vi "Report Loop.vi"(8 "error in (no error)":errorcluster) -> (0 "error out":errorcluster)   [LabVIEW 2020, in "Report.lvlib"]
doc: "Message loop for handling messages pertaining to the acquisition of data from the hardware."
uses:
  Report.lvlib
  support/PCT FGV CMD.ctl
  REP Configuration.ctl
  Test Setting.ctl
  Acquisition State.ctl
  support/Message Queue/Enqueue Message (Single).vi
  <vilib>/Utility/error.llb/Error Cluster From Error Code.vi
  <vilib>/ErrorRing/Error Ring.xnode
  support/Message Queue/Message Queue.lvlib
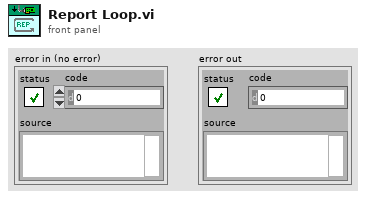
[diagram p1: front panel]
types:
  T1 = typedef "PCT FGV CMD.ctl" = enum16{"INIT", "GET", "SET"}
  T2 = typedef "Message Queue.lvlib/All Message Queues.ctl" = cluster{"UI":refnum<queue>, "Logging":refnum<queue>, "LOG":refnum<queue>, "ALARM":refnum<queue>, "Test":refnum<queue>, "Answer":refnum<queue>, "PLC":refnum<queue>, "DB":refnum<queue>, "Report":refnum<queue>, "OPC":refnum<queue>, "Procedure":refnum<queue>, "PalmSens":refnum<queue>, "SYS 7000 Reader":refnum<queue>, "SWITCH":refnum<queue>, "MOTOR":refnum<queue>, "MOTION":refnum<queue>, "HIDEN":refnum<queue>, "VALVE":refnum<queue>, "MFC":refnum<queue>, "PUMP IN":refnum<queue>, "PUMP OUT":refnum<queue>}
  T3 = typedef "Report.lvlib/REP Configuration.ctl" = cluster{"Test Setting":T4, "Measurements":string[][], "LOG REF":refnum<vi>, "Report Template":path, "Save Report path":path, "Data File Path":path, "Popup Dialog":bool}
  T4 = typedef "Report.lvlib/Test Setting.ctl" = cluster{"Test_Num":i32, "Test_ID":i32, "Proc_ID":i32, "Max Force":dbl, "User":string, "SN":string, "Date":string}
  T5 = typedef "Report.lvlib/Acquisition State.ctl" = enum16{"Idle", "Acquiring"}
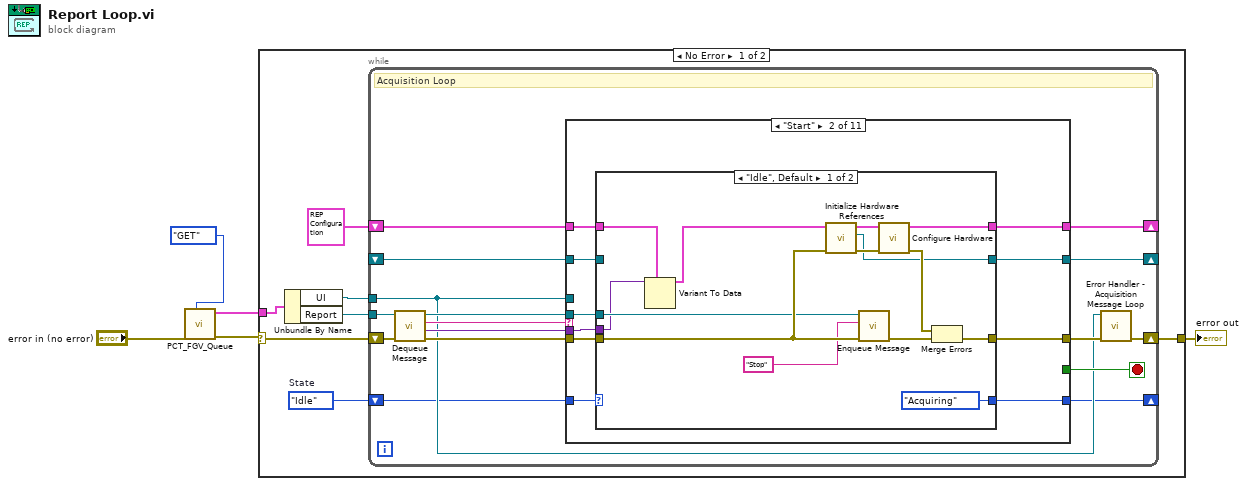
[diagram p0: block diagram]
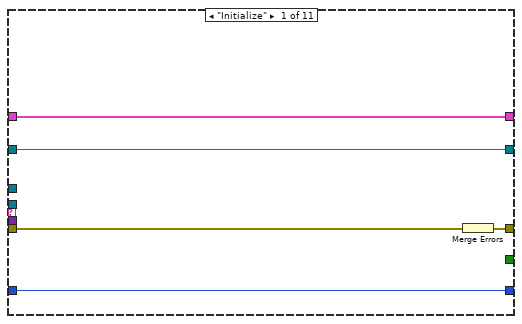
[diagram p2: hidden frame]
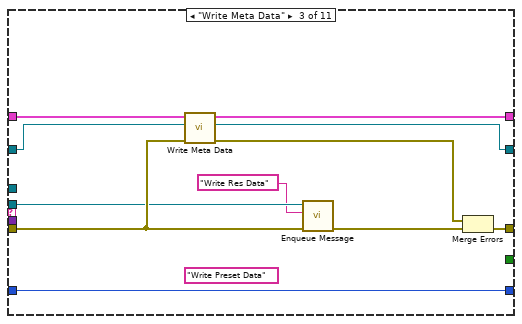
[diagram p4: hidden frame]
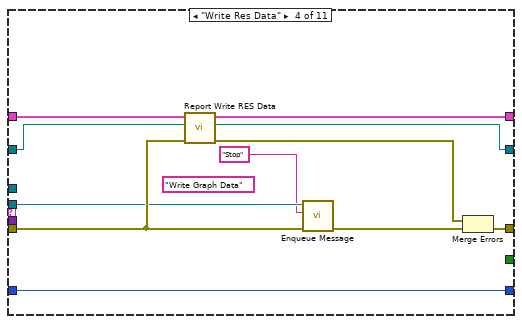
[diagram p5: hidden frame]
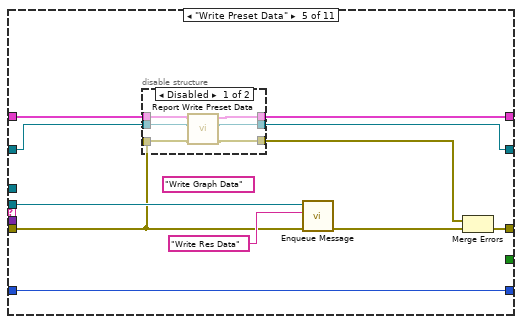
[diagram p6: hidden frame]
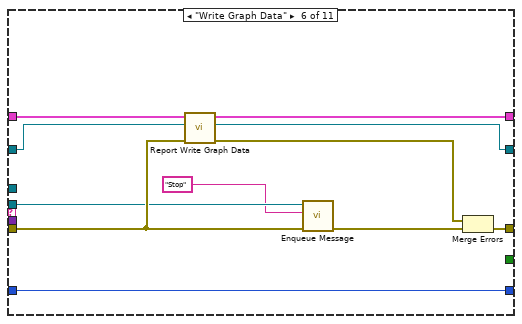
[diagram p8: hidden frame]
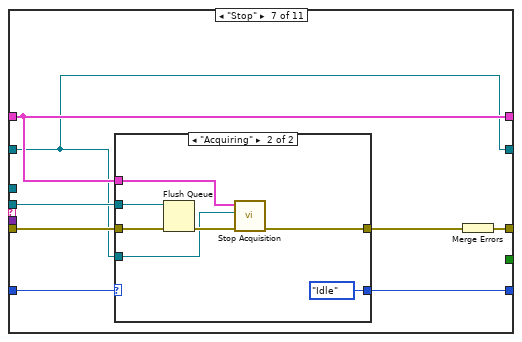
[diagram p9: hidden frame]
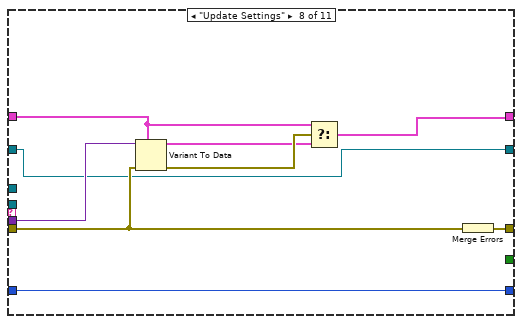
[diagram p11: hidden frame]
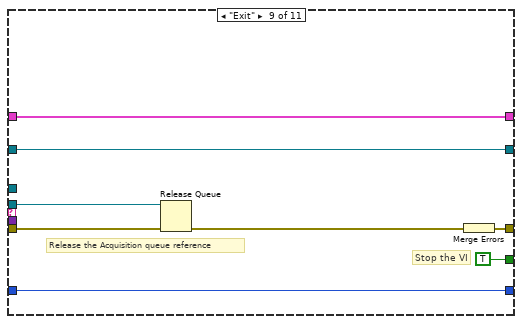
[diagram p12: hidden frame]
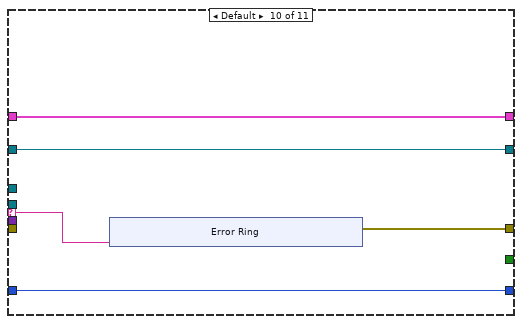
[diagram p13: hidden frame]
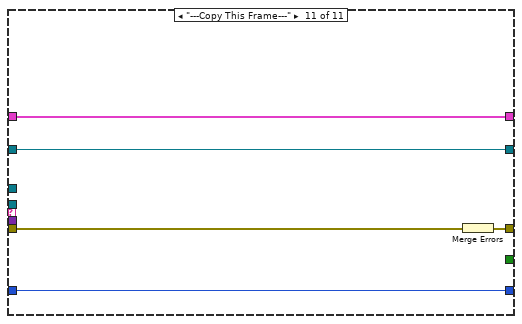
[diagram p14: hidden frame]
diagram:
  n1 = call "PCT_FGV_Queue.vi"("CMD"=PCT_FGV_CMD."GET", "error in (no error)"="error in (no error)") -> ("error out"=w3:errorcluster, "Message Queues out"=w2:T2)  [unwired: 8 in]
  n2 = case shown="No Error" w3 {
    selector: w3 -> [w8 w165]
    tunnel: w2 -> [w12 _]
    tunnel: [w10 w165] -> w5
    frame No Error {
      w6 = Acquisition_State."Idle"  # State
      n3 = Unbundle By Name(w12) -> ("UI"=w7:refnum<queue>, "Report"=w11:refnum<queue>)
      n4 = while {
        tunnel: w11 -> [w20]
        shift-right: [w27] -> _
        shift-left: T3 {"Test Setting"={"Test_Num"=0, "Test_ID"=0, "Proc_ID"=0, "Max Force"=0.0, "User"="", "SN"="", "Date"=""}, "Measurements"=[[""]], "LOG REF"=refnum, "Report Template"=path "", "Save Report path"=path "", "Data File Path"=path "", "Popup Dialog"=FALSE} ("Data Cluster") -> [w28]
        shift-right: [w18] -> w10
        shift-left: w8 -> [w25]
        tunnel: w7 -> [w17]
        shift-right: [w15] -> _
        shift-left: w6 -> [w16]
        shift-right: [w14] -> _
        shift-left: _ -> [w13]
        stop <- w26 stop-if-true
        # "Acquisition Loop"
        n5 = call "Dequeue Message.vi"("error in (no error)"=w25, "Message Queue"=w20) -> ("error out"=w24:errorcluster, "Message Data"=w22:variant, "Message"=w23:string, "dup Message Queue"=w21:refnum<queue>)  [unwired: 6 in]
        n6 = case "Message Cases" shown="\"Start\"" w23 {
          selector: w23 -> [_ _ _ _ _ _ _ _ _ w151 _]
          tunnel: w21 -> [_ w37 w65 w76 w91 w106 w118 _ w143 _ _]
          tunnel: w24 -> [w32 w41 w67 w78 w85 w108 w120 w133 w145 _ w164]
          tunnel: [w33 w43 w72 w83 w94 w113 w121 w139 w146 w150 w162] -> w19
          tunnel: w28 -> [w31 w42 w69 w80 w89 w110 w119 w135 w142 w152 w163]
          tunnel: [w31 w40 w70 w81 w88 w111 w119 w134 w142 w152 w163] -> w27
          tunnel: [_ _ _ _ _ _ _ _ TRUE _ _] -> w26
          tunnel: w22 -> [_ w36 _ _ _ _ _ w138 _ _ _]
          tunnel: w17 -> [_ _ _ _ _ _ _ _ _ _ _]
          tunnel: w16 -> [w30 w39 w68 w79 w93 w109 w117 w132 w141 w149 w161]
          tunnel: [w30 w38 w68 w79 w93 w109 w116 w132 w141 w149 w161] -> w15
          tunnel: [w29 w35 w63 w74 w87 w103 w114 w131 w140 w148 w160] -> w14
          tunnel: w13 -> [w29 w34 w64 w75 w86 w104 w114 w131 w140 w148 w160]
          frame "Initialize" {
            # "Initialize  - Initialize is currently a no-op.  The hardware initialization takes place in the 'Start' message."
            n7 = Merge Errors(w32) -> (w33:errorcluster)
          }
          frame "Start" {
            # "Start - Configure and start the acquisition."
            n8 = case shown="\"Idle\", Default" w39 {
              selector: w39 -> [_ w59]
              tunnel: [w57 w61] -> w43
              tunnel: w42 -> [w45 w60]
              tunnel: w41 -> [w51 w61]
              tunnel: [w53 w60] -> w40
              tunnel: [Acquisition_State."Acquiring" ("State") w59] -> w38
              tunnel: w37 -> [w49 _]
              tunnel: w36 -> [w47 _]
              tunnel: [w46 w58] -> w35
              tunnel: w34 -> [_ w58]
              frame "Idle", Default {
                # "If the system is idle, start the acquisition."
                n9 = Variant To Data(type=w45, Variant=w47) -> (data=w44:T3)  [unwired: 1 in, 1 out]
                n10 = call "Initialize Hardware References.vi"("error in (no error)"=w51, "Hardware Resources in"=w44) -> ("error out"=w56:errorcluster, "report out"=w46:refnum<class "NI_report.lvclass">, "Hardware Resources out"=w54:T3)  [unwired: 7 in]
                n11 = call-poly "Enqueue Message.vi"("error in (no error)"=w51, "Message"="Stop", "Message Queue"=w49) -> ("error out"=w50:errorcluster)  [unwired: 7 in, 1 out]
                n12 = call "Configure Hardware.vi"("error in (no error)"=w56, "Hardware Resources in"=w54) -> ("error out"=w55:errorcluster, "Hardware Resources out"=w53:T3)  [unwired: 8 in]
                n13 = Merge Errors(w55, w50) -> (w57:errorcluster)
              }
              frame "Acquiring" {
                # "The system is already acquiring. Ignore the \"Start\" message."
              }
            }
          }
          frame "Write Meta Data" {
            (unwired) "Write Preset Data"
            # "Acquire - Acquire data from the hardware. Since this is a continuous acquisition, this message will always message itself to run again."
            n14 = call "Write Meta Data.vi"("error in (no error)"=w67, "report in"=w64, "Hardware Resources in"=w69) -> ("error out"=w71:errorcluster, "report out"=w63:refnum<class "NI_report.lvclass">, "Hardware Resources out"=w70:T3)  [unwired: 6 in]
            n15 = call-poly "Enqueue Message.vi"("error in (no error)"=w67, "Message"="Write Res Data", "Message Queue"=w65) -> ("error out"=w66:errorcluster)  [unwired: 7 in, 1 out]
            n16 = Merge Errors(w71, w66) -> (w72:errorcluster)
          }
          frame "Write Res Data" {
            (unwired) "Write Graph Data"
            # "Acquire - Acquire data from the hardware. Since this is a continuous acquisition, this message will always message itself to run again."
            n17 = call "Report Write RES Data.vi"("error in (no error)"=w78, "report in"=w75, "Hardware Resources in"=w80) -> ("error out"=w82:errorcluster, "report out"=w74:refnum<class "NI_report.lvclass">, "Hardware Resources out"=w81:T3)  [unwired: 6 in]
            n18 = call-poly "Enqueue Message.vi"("error in (no error)"=w78, "Message"="Stop", "Message Queue"=w76) -> ("error out"=w77:errorcluster)  [unwired: 7 in, 1 out]
            n19 = Merge Errors(w82, w77) -> (w83:errorcluster)
          }
          frame "Write Preset Data" {
            (unwired) "Write Graph Data"
            # "Acquire - Acquire data from the hardware. Since this is a continuous acquisition, this message will always message itself to run again."
            n20 = disable-structure shown="Disabled" {
              disable-tunnel: w89 -> [w100 w102]
              disable-tunnel: [w99 w102] -> w88
              disable-tunnel: [w98 w101] -> w87
              disable-tunnel: w86 -> [w97 w101]
              disable-tunnel: w85 -> [w96 _]
              disable-tunnel: [w95 _] -> w84
              frame Disabled {
                n21 = call "Report Write Preset Data.vi"("error in (no error)"=w96, "report in"=w97, "Hardware Resources in"=w100) -> ("error out"=w95:errorcluster, "report out"=w98:refnum<class "NI_report.lvclass">, "Hardware Resources out"=w99:T3)  [unwired: 6 in]
              }
              frame Enabled {
              }
            }
            n22 = call-poly "Enqueue Message.vi"("error in (no error)"=w85, "Message"="Write Res Data", "Message Queue"=w91) -> ("error out"=w92:errorcluster)  [unwired: 7 in, 1 out]
            n23 = Merge Errors(w84, w92) -> (w94:errorcluster)
          }
          frame "Write Graph Data" {
            # "Acquire - Acquire data from the hardware. Since this is a continuous acquisition, this message will always message itself to run again."
            n24 = call "Report Write Graph Data.vi"("error in (no error)"=w108, "report in"=w104, "Hardware Resources in"=w110) -> ("error out"=w112:errorcluster, "report out"=w103:refnum<class "NI_report.lvclass">, "Hardware Resources out"=w111:T3)  [unwired: 6 in]
            n25 = call-poly "Enqueue Message.vi"("error in (no error)"=w108, "Message"="Stop", "Message Queue"=w106) -> ("error out"=w107:errorcluster)  [unwired: 7 in, 1 out]
            n26 = Merge Errors(w112, w107) -> (w113:errorcluster)
          }
          frame "Stop" {
            # "Stop - Stop the Acquisition. Also flush the queue of any pending \"Acquire\" messages."
            n27 = case shown="\"Acquiring\"" w117 {
              selector: w117 -> [w123 _]
              tunnel: w120 -> [w122 w130]
              tunnel: w119 -> [_ w129]
              tunnel: w118 -> [_ w127]
              tunnel: [w123 Acquisition_State."Idle" ("State")] -> w116
              tunnel: [w122 w125] -> w115
              tunnel: w114 -> [_ w124]
              frame "Idle", Default {
                # "The system is already idle. Ignore the \"Stop\" message."
              }
              frame "Acquiring" {
                # "If the system is acquiring, stop the acquisition."
                n28 = Flush Queue(queue=w127, error in (no error)=w130) -> (error out=w128:errorcluster)  [unwired: 2 out]
                n29 = call "Stop Acquisition.vi"("error in (no error)"=w128, "report in"=w124, "Hardware Resources in"=w129) -> ("error out"=w125:errorcluster)  [unwired: 8 in]
              }
            }
            n30 = Merge Errors(w115) -> (w121:errorcluster)
          }
          frame "Update Settings" {
            # "New settings are available, update the current ones stored in the shift register with the settings sent as part of the message"
            n31 = Variant To Data(error in=w133, type=w135, Variant=w138) -> (data=w136:T3, error out=w137:errorcluster)
            n32 = Select(t=w135, s=w137, f=w136) -> (s? t:f=w134:T3)
            n33 = Merge Errors(w133) -> (w139:errorcluster)
          }
          frame "Exit" {
            # "Release the Acquisition queue reference"
            # "Stop the VI"
            # "Exit - Send the Exit message to the UI Message Handler."
            n34 = Release Queue(queue=w143, error in (no error)=w145) -> (error out=w144:errorcluster)  [unwired: 1 in, 2 out]
            n35 = Merge Errors(w144) -> (w146:errorcluster)
          }
          frame Default {
            # "'Default' case only runs if there is a message that isn't defined in any of the other cases.  Output a programming error."
            n36 = xnode "Error Ring"("parameter 0"=w151) -> ("error out"=w150:errorcluster)
          }
          frame "---Copy This Frame---" {
            # "Duplicate this frame when creating new messages.  Change this comment in the duplicated frame to describe this message."
            n37 = Merge Errors(w164) -> (w162:errorcluster)
          }
        }
        n38 = call "Error Handler - Acquisition Message Loop.vi"("error in (no error)"=w19, "Message Queue"=w17) -> ("dup error in"=w18:errorcluster)  [unwired: 8 in, 1 out]
      }
    }
    frame Error {
    }
  }
  "error out" <- w5
